vi "libssh2_userauth_password_ex.vi"(7 "passwd_change_cb":u64, 8 "error in (no error)":errorcluster, 9 "password":string, 10 "username":string, 11 "session":T1) -> (0 "error out":errorcluster, 3 "return value":i32)   [LabVIEW 2013, in "libssh2.lvlib"]
doc: "Authenticates a session with username and password."
uses:
  libssh2.lvlib
  Session Refnum.ctl
  libssh2.dll
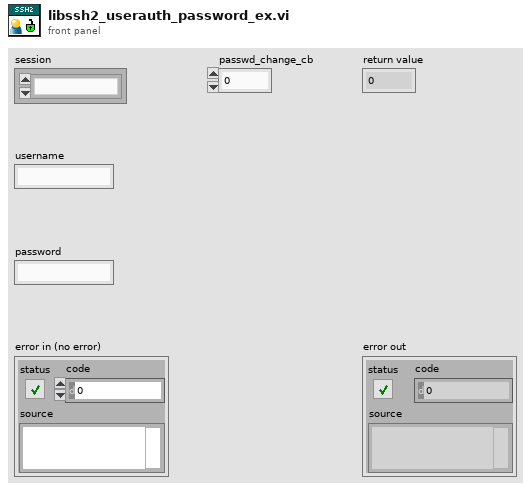
[diagram p1: front panel]
types:
  T1 = typedef "libssh2.lvlib/Session Refnum.ctl" = refnum<k1>
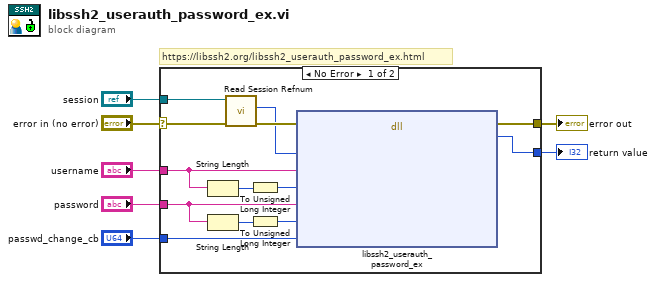
[diagram p0: block diagram]
diagram:
  # "https://libssh2.org/libssh2_userauth_password_ex.html"
  n1 = case shown="No Error" "error in (no error)" {
    selector: "error in (no error)" -> [w8 w21]
    tunnel: "username" -> [w20 _]
    tunnel: "password" -> [w18 _]
    tunnel: "passwd_change_cb" -> [w16 _]
    tunnel: [w15 _] -> w4
    tunnel: [w14 w21] -> w3
    tunnel: "session" -> [w10 _]
    frame No Error {
      n2 = String Length(string=w20) -> (length=w12:i32)
      n3 = String Length(string=w18) -> (length=w13:i32)
      n4 = call "Read Session Refnum.vi"("error in (no error)"=w8, "session"=w10) -> ("error out"=w11:errorcluster, "LIBSSH2_SESSION*"=w9:u64)  [unwired: 8 in]
      n5 = To Unsigned Long Integer(number=w12) -> (unsigned 32bit integer=w19:u32)
      n6 = To Unsigned Long Integer(number=w13) -> (unsigned 32bit integer=w17:u32)
      n7 = dll-call lib="C:/Users/pasca/source/repos/libssh2-labview/libssh2**.*" fn="libssh2_userauth_password_ex"(error in=w11, "session"=w9, "username"=w20, "username_len"=w19, "password"=w18, "password_len"=w17, "passwd_change_cb"=w16) -> (error out=w14:errorcluster, "return value"=w15:i32)  [unwired: 8 in, 1 out]
    }
    frame Error {
    }
  }
  "return value" <- w4
  "error out" <- w3
